vi "Hardware Device Get All Info.vi"(8 "error in":errorcluster, 11 "NI Analog Input in":refnum<class "NI Analog Input.lvclass">) -> (0 "error out":errorcluster, 3 "NI Analog Input out":refnum<class "NI Analog Input.lvclass">)   [LabVIEW 2023, in "HardwareAbstractionLayer_LVOOP.lvlib" / "NI Analog Input.lvclass"]
doc: "This VI is AI Physical Channel Read"
uses:
  NI Analog Input.lvclass
  NI Analog Input.lvclass/NI Analog Input.ctl
  <resource>/objmgr/daqmx.rc
panel:
  out "AI.PhysicalChans":tag[](array[tag])
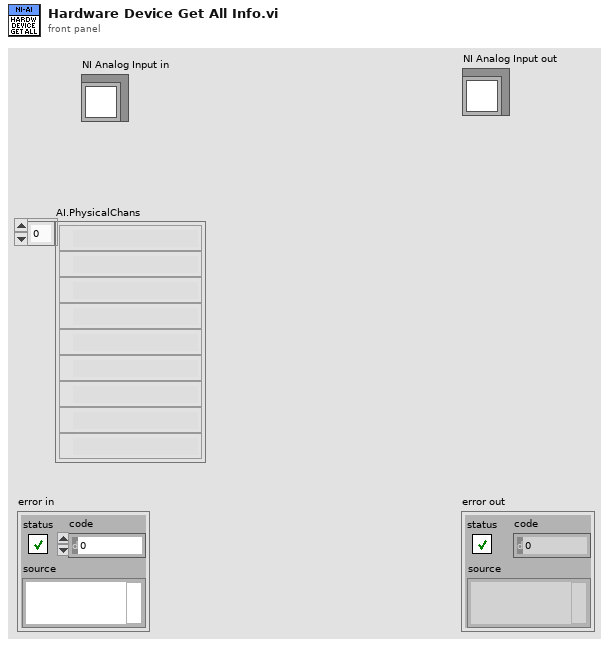
[diagram p1: front panel]
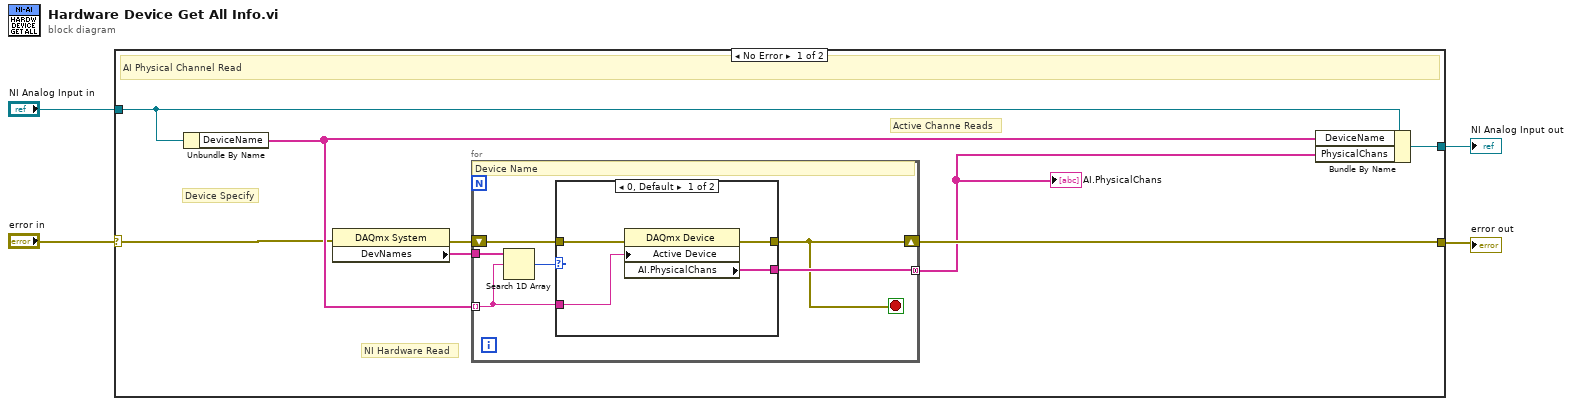
[diagram p0: block diagram]
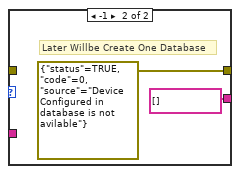
[diagram p2: hidden frame]
diagram:
  n1 = case shown="No Error" "error in" {
    selector: "error in" -> [w7 w26]
    tunnel: [w6 w26] -> w3
    tunnel: [w12 w25] -> w1
    tunnel: "NI Analog Input in" -> [w11 w25]
    frame No Error {
      # "Active Channe Reads"
      # "Device Specify"
      # "NI Hardware Read"
      # "AI Physical Channel Read"
      n2 = Unbundle By Name(w11) -> ("DeviceName"=w10:tag[])
      n3 = property class="DAQmx System"(error in=w7) -> (error out=w8:errorcluster, "DevNames"=w9:tag[])  [unwired: 1 in, 1 out]
      n4 = for {
        tunnel: w10 -> [w15] mode=indexing
        tunnel: w9 -> [w16]
        tunnel: [w14] -> w5 mode=concatenating
        shift-right: [w13] -> w6
        shift-left: w8 -> [w17]
        stop <- w13 stop-if-true
        # "Device Name"
        n5 = Search 1D Array(1D array=w16, element=w15) -> (index of element=w18:i32)  [unwired: 1 in]
        n6 = case shown="0, Default" w18 {
          tunnel: w17 -> [w20 _]
          tunnel: [w19 errorcluster {"status"=TRUE, "code"=0, "source"="Device  Configured in database is not avilable"} ("error out")] -> w13
          tunnel: w15 -> [w22 _]
          tunnel: [w21 tag[] [] ("AI.PhysicalChans")] -> w14
          frame 0, Default {
            n7 = property class="DAQmx Device"(error in=w20, "Active Device"=w22) -> (error out=w19:errorcluster, "AI.PhysicalChans"=w21:tag[])  [unwired: 1 in, 1 out]
          }
          frame -1 {
            # "Later Willbe Create One Database"
          }
        }
      }
      "AI.PhysicalChans" <- w5
      n8 = Bundle By Name(cluster=w11, "DeviceName"=w10, "PhysicalChans"=w5) -> (w12:refnum<class "NI Analog Input.lvclass">)
    }
    frame Error {
    }
  }
  "error out" <- w3
  "NI Analog Input out" <- w1
